vi "get poisition.vi"(6 "error in (no error)":errorcluster, 7 "Instrument Ref In":refnum<k24>) -> (1 "Position":dbl, 2 "error out":errorcluster, 3 "Instrument Ref Out 2":refnum<k24>)   [LabVIEW 2019, in "SubVI.lvlib"]
uses:
  SubVI.lvlib
  C:/Users/618/Desktop/measure/lib/QDInstrument.dll
  lib/QDInstrument.dll
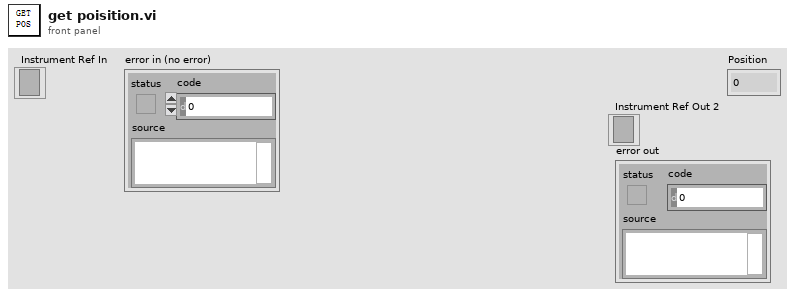
[diagram p1: front panel]
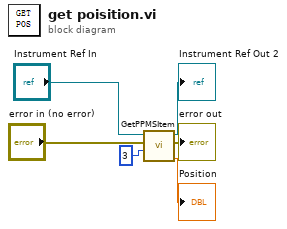
[diagram p0: block diagram]
diagram:
  n1 = call "GetPPMSItem.vi"("Channel"=3, "error in (no error)"="error in (no error)", "Instrument Ref In"="Instrument Ref In") -> ("Result"=→"Position":dbl, "error out"=→"error out":errorcluster, "Instrument Ref Out"=→"Instrument Ref Out 2":refnum<k24>)  [unwired: 1 in, 1 out]
